vi "setSignal.vi"(0 "reference":refnum<class "CallEdge.lvclass">, 1 "signal":bool, 5 "error in (no error)":errorcluster) -> (14 "reference out":refnum<class "CallEdge.lvclass">, 19 "error out":errorcluster)   [LabVIEW 2016, in "CallEdge.lvclass"]
doc: "public void setSignal(boolean newValue)"
uses:
  <resource>/Framework/Providers/Open_GDS/UML/CallEdge_class/CallEdge.lvclass
  <resource>/Framework/Providers/Open_GDS/UML/ArrowHead_class/ArrowHeadType.ctl
  <resource>/Framework/Providers/Open_GDS/UML/ArrowHead_class/ArrowHead.lvclass
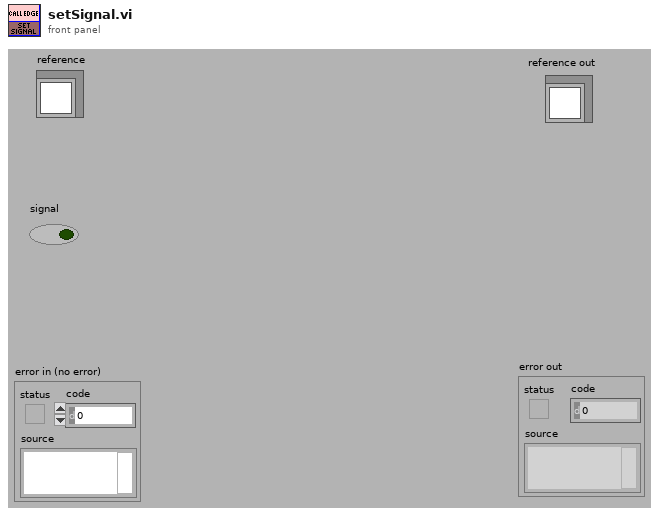
[diagram p1: front panel]
types:
  T1 = typedef "ArrowHead.lvclass/ArrowHeadType.ctl" = enum16{"NONE", "TRIANGLE", "BLACK_TRIANGLE", "V", "HALF_V", "DIAMOND", "BLACK_DIAMOND"}
  T2 = typedef "CallEdge.lvclass/ObjectAttributes.ctl" = cluster{"signal":bool}
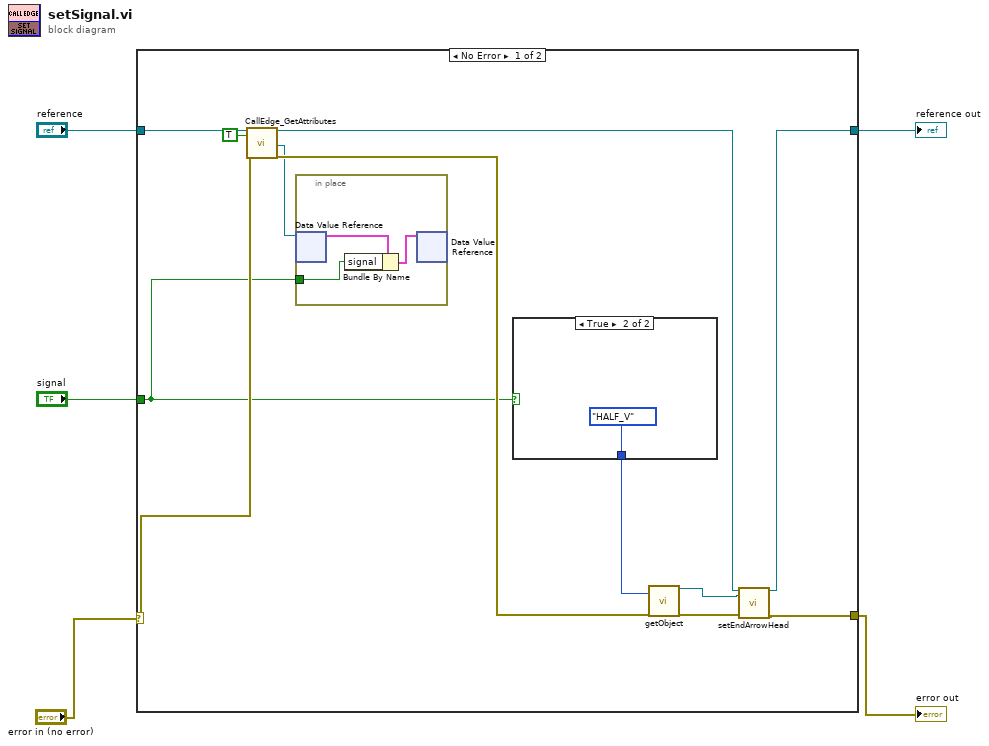
[diagram p0: block diagram]
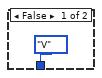
[diagram p2: hidden frame]
diagram:
  n1 = case shown="No Error" "error in (no error)" {
    selector: "error in (no error)" -> [w14 w23]
    tunnel: "reference" -> [w17 w24]
    tunnel: [w16 w23] -> w4
    tunnel: [w15 w24] -> w3
    tunnel: "signal" -> [w6 _]
    frame No Error {
      n2 = call <resource>:"CallEdge_GetAttributes.vi"("reference in"=w17, "OnlyGetDvrReference(False)"=TRUE, "error in (no error)"=w14) -> ("reference out"=w9:refnum<class "CallEdge.lvclass">, "DataRef"=w7:refnum<data-value>, "error out"=w11:errorcluster)  [unwired: 13 in, 1 out]
      n3 = in-place {
        in-place-border: w6 -> [w19]
        n4 = in-place-dvr #1(w7) -> (w20:T2)  [unwired: 1 out]
        n5 = Bundle By Name(cluster=w20, "signal"=w19) -> (w18:T2)
        n6 = in-place-dvr #1(w18) -> ()  [unwired: 2 out]
      }
      n7 = case shown="True" w6 {
        tunnel: [ArrowHeadType."V" ("arrowHead") ArrowHeadType."HALF_V" ("arrowHead")] -> w10
        frame False {
        }
        frame True {
        }
      }
      n8 = call <resource>:"getObject.vi"("arrowHead"=w10, "error in (no error)"=w11) -> ("reference out"=w12:refnum<class "ArrowHead.lvclass">, "error out"=w13:errorcluster)  [unwired: 16 out]
      n9 = call-dynamic "setEndArrowHead.vi"("reference"=w9, "endArrowHead"=w12, "error in (no error)"=w13) -> ("reference out"=w15:refnum<class "CallEdge.lvclass">, "error out"=w16:errorcluster)  [unwired: 15 out]
    }
    frame Error {
    }
  }
  "reference out" <- w3
  "error out" <- w4
